vi "4011_12_13_14_16_get_rdg.vi"(0 "Address":T1, 1 "Channel Name":string) -> (3 "Comment":string, 5 "Reading":dbl format="%.3f")   [LabVIEW 2010]
uses:
  ADAM Client/Sub VIs/ADAM Controls/Address.ctl
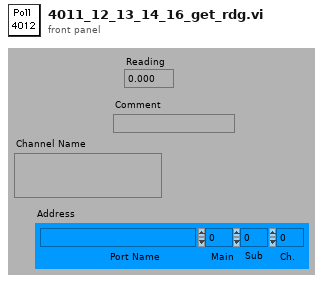
[diagram p1: front panel]
types:
  T1 = typedef "Address.ctl" = cluster{"Main":i32, "Ch.":i32, "Sub":i32, "Port Name":string}
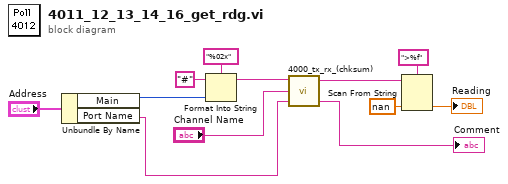
[diagram p0: block diagram]
diagram:
  n1 = Unbundle By Name("Address") -> ("Main"=w2:i32, "Port Name"=w1:string)
  n2 = Format Into String(format string="%02x", initial string="#", w2) -> (resulting string=w10:string)  [unwired: 1 in, 1 out]
  n3 = call "4000_tx_rx_(chksum).vi"("Port Name"=w1, "Channel Name"="Channel Name", "Write String"=w10) -> ("Comment out"=→"Comment":string, "Read"=w8:string)  [unwired: 1 out]
  n4 = Scan From String(format string=">%f", input string=w8, default 1=nan ("Reading")) -> (output 1=→"Reading":dbl)  [unwired: 2 in, 3 out]
